vi "Complex Cholesky Factorization.vi"(0 "A":T1) -> (1 "Cholesky R":T1, 2 "error":i32)   [LabVIEW 2010, in "NI_AALPro.lvlib"]
doc: "Performs Cholesky factorization on a symmetric or Hermitian positive definite matrix. Wire data to the <B>A</B> input to determine the polymorphic instance to use or manually select the instance."
uses:
  NI_AALPro.lvlib
  ComplexMatrix.ctl
  NI_AALBase.lvlib
  NI_Matrix.lvlib
panel:
  # "Complex Cholesky Factorization"
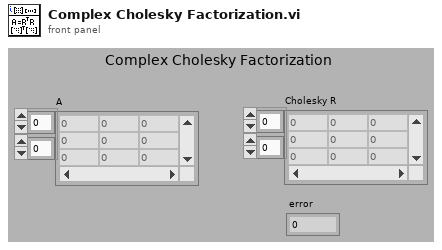
[diagram p1: front panel]
types:
  T1 = typedef "NI_Matrix.lvlib/ComplexMatrix.ctl" = cdb[][]
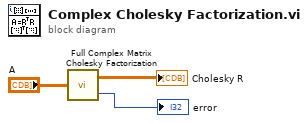
[diagram p0: block diagram]
diagram:
  n1 = call "Full Complex Matrix Cholesky Factorization.vi"("A"="A") -> ("Cholesky R"=→"Cholesky R":T1, "error"=→"error":i32)
